vi "ROS_Topic_Write.vi"(2 "Msg in":string, 3 "Continuous?":bool, 4 "ROS in":T1) -> (1 "ROS out":T1)   [LabVIEW 2013]
doc: "Prepends the length to Msg in before sending out the data on the specified topic. Use only for publishers and service clients. Messages need to be formatted using Message Building functionality. \n\nSetting Continuous to True will instruct the server to publish the message it received as quickly as possible, updating the message when a new ROS_Topic_Write is called."
uses:
  SubVIs/_ROSControl.ctl
  SubVIs/_ROSDirection.ctl
panel:
  out "msg out (HEX)":string
  out "msg out":string
  # "9800 0000 0100 0000 0700 0000 6573\n2D38 52C1 E0BF A915 A15D DEEC EBBF\n0000 0000 0000 0000 182D 4454 FB21 \nE93F 0000 0000 0000 0000 61A1 F2D8 \n6C87 FA3F 0000 0000 0000 0000 0700 \n0000 0800 0000 7269 6768 745F 7330 \n0800 0000 7269 6768 745F 7331 0800 \n0000 7269 6768 745F 6530 0800 0000 \n7269 6768 745F 6531 0800 0000 7269 \n6768 745F 7730 0800 0000 7269 6768 \n745F 7731 0800 0000 7269 6768 745F \n7732"
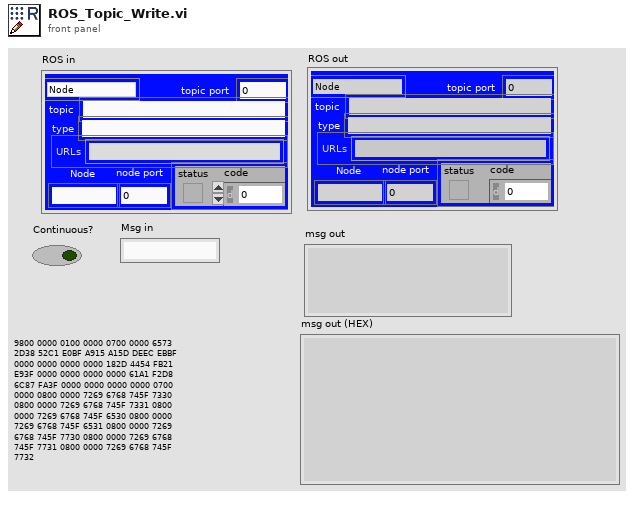
[diagram p1: front panel]
types:
  T1 = typedef "_ROSControl.ctl" = cluster{"topic port":u16, "Node":string, "topic":string, "type":string, "node port":u32, "error ":errorcluster, "Direction":T2, "APIs":string[]}
  T2 = typedef "_ROSDirection.ctl" = enum16{"Node", "Publisher", "Subscriber", "Service Client"}
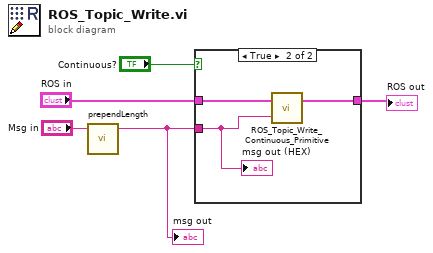
[diagram p0: block diagram]
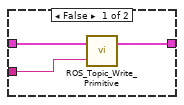
[diagram p2: hidden frame]
diagram:
  n1 = call "prependLength.vi"("msg in"="Msg in") -> ("msg out"=w1:string)  [unwired: 4 in]
  "msg out" <- w1
  n2 = case shown="True" "Continuous?" {
    tunnel: "ROS in" -> [w8 w11]
    tunnel: [w7 w10] -> w4
    tunnel: w1 -> [w6 w9]
    frame False {
      n3 = call "ROS_Topic_Write_Primitive.vi"("Msg in"=w6, "ROS in"=w8) -> ("ROS out"=w7:T1)  [unwired: 1 in]
    }
    frame True {
      n4 = call "ROS_Topic_Write_Continuous_Primitive.vi"("Msg in"=w9, "ROS in"=w11) -> ("ROS out"=w10:T1)  [unwired: 1 in]
      "msg out (HEX)" <- w9
    }
  }
  "ROS out" <- w4
